vi "increment.vi"() -> ()   [LabVIEW 2015]
panel:
  out "x .and. y?":bool
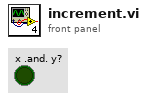
[diagram p1: front panel]
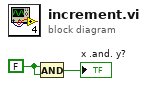
[diagram p0: block diagram]
diagram:
  w2 = FALSE ("x")
  n1 = And(x=w2, y=w2) -> (x .and. y?=→"x .and. y?":bool)
